vi "精度判定.vi"(8 "精度":dbl, 9 "零飘":dbl, 10 "实际电流":dbl[](array[numeric]), 11 "报文数组":string[][](array[string])) -> (2 "判定":bool[](array[boolean]), 3 "误差":dbl[](array[numeric]))   [LabVIEW 2021]
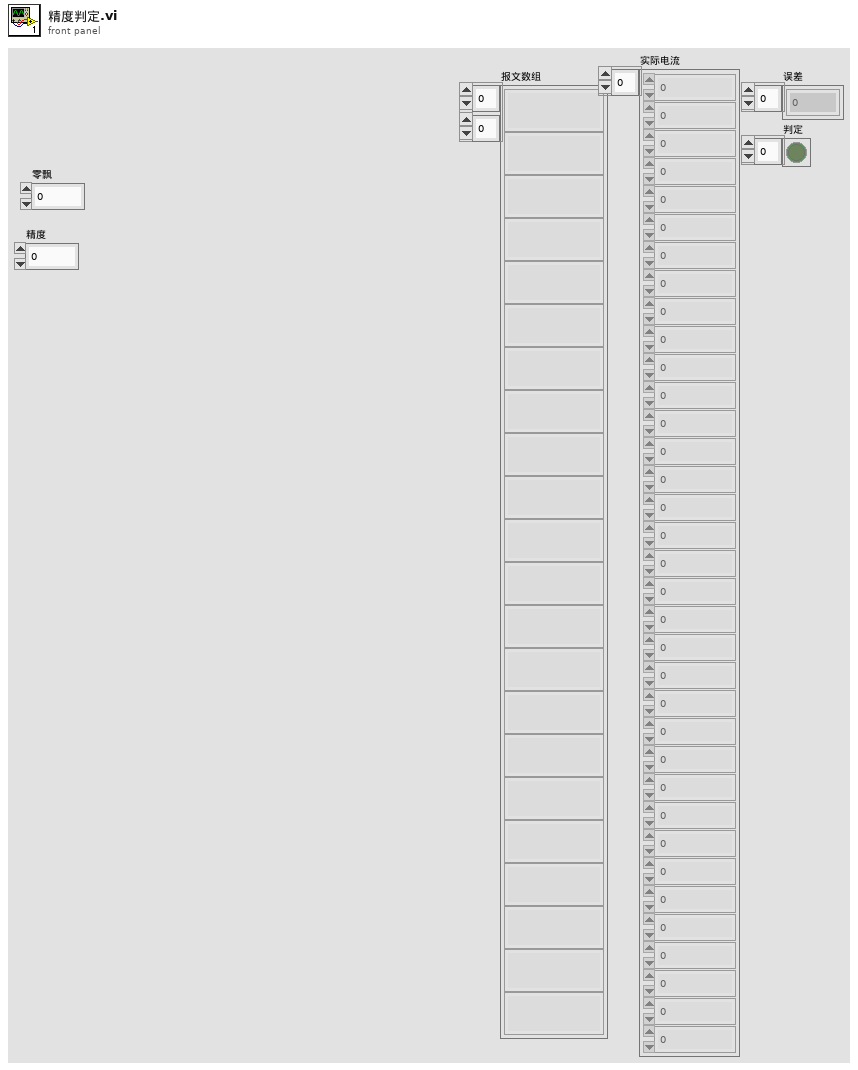
[diagram p1: front panel]
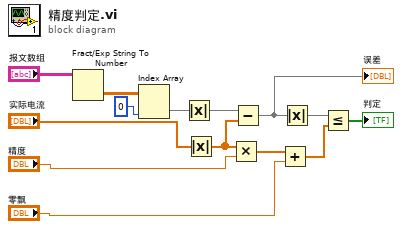
[diagram p0: block diagram]
diagram:
  n1 = Fract/Exp String To Number(string="报文数组") -> (number=w14:dbl[][])  [unwired: 3 in, 1 out]
  n2 = Index Array(array=w14, index (col)=0 ("禁用的索引 (列)")) -> (element=w11:dbl[])  [unwired: 1 in]
  n3 = Absolute Value(x=w11) -> (abs(x)=w9:dbl[])
  n4 = Absolute Value(x="实际电流") -> (abs(x)=w7:dbl[])
  n5 = Multiply(x=w7, y="精度") -> (x*y=w6:dbl[])
  n6 = Subtract(x=w9, y=w7) -> (x-y=w8:dbl[])
  "误差" <- w8
  n7 = Add(x=w6, y="零飘") -> (x+y=w4:dbl[])
  n8 = Absolute Value(x=w8) -> (abs(x)=w5:dbl[])
  n9 = Less Or Equal?(x=w5, y=w4) -> (x <= y?=→"判定":bool[])
